vi "test_FHWM.vi"() -> ()   [LabVIEW 2010]
uses:
  <userlib>/gfitsio/cfitsio-bitpix.ctl
  <userlib>/gfitsio/gfitsio-write-image-subset-sgl-2d.vi
  <userlib>/gfitsio/gfitsio.lvlib
panel:
  out "standard error":string
  out "standard output":string
  out "Y FWHM":dbl
  out "X FWHM":dbl
  in  "file path":path
  in  "GuidingStar":i32[][](graph)=[[309, 321, 390, 345, 402, 429, 369, 350, 376, 446, 351, 379, 352, 433, 465, 428, 405, 434, 390, 451, 355, 427, 455, 373, 373, 382, 407, 375, 357, 334, 281, 423], [362, 320, 373, 482, 385, 392, 364, 408, 398, 394, 436, 441, 484, 430, 505, 486, 452, 396, 448, 421, 415, 430, 363, 393, 473, 365, 337, 363, 396, 352, 342, 314], [417, 380, 414, 379, 438, 403, 518, 467, 469, 542, 514, 462, 541, 513, 503, 478, 546, 555, 525, 534, 510, 508, 452, 452, 440, 497, 425, 460, 378, 384, 437, 370], [291, 408, 345, 406, 406, 391, 490, 415, 451, 464, 469, 482, 479, 592, 534, 617, 582, 651, 534, 608, 533, 546, 502, 464, 481, 420, 401, 426, 427, 369, 365, 381], [444, 344, 357, 415, 447, 451, 389, 456, 410, 560, 515, 560, 540, 611, 640, 660, 653, 638, 654, 635, 619, 553, 506, 527, 537, 482, 443, 526, 380, 421, 412, 352], [413, 430, 389, 460, 469, 502, 481, 483, 501, 532, 660, 673, 737, 685, 795, 855, 831, 938, 738, 816, 711, 705, 655, 550, 547, 517, 518, 434, 467, 475, 439, 435], [391, 342, 490, 394, 485, 498, 494, 539, 569, 614, 630, 793, 834, 856, 956, 973, 1101, 1011, 1042, 957, 865, 766, 732, 684, 680, 584, 533, 564, 478, 598, 410, 456], [365, 340, 405, 510, 514, 534, 516, 661, 656, 691, 754, 885, 987, 1132, 1170, 1267, 1305, 1364, 1216, 1278, 993, 973, 841, 883, 741, 564, 579, 490, 590, 501, 440, 451], [409, 405, 430, 463, 544, 553, 603, 650, 765, 840, 906, 1134, 1123, 1399, 1536, 1694, 1650, 1728, 1711, 1528, 1303, 1170, 997, 877, 919, 738, 659, 669, 591, 596, 483, 514], [456, 469, 513, 505, 489, 589, 638, 769, 803, 945, 1114, 1345, 1566, 1679, 1933, 2132, 2273, 2098, 2068, 1908, 1615, 1462, 1274, 1103, 1003, 911, 787, 650, 626, 608, 543, 474], [553, 456, 508, 563, 632, 676, 833, 854, 1011, 1212, 1417, 1611, 1915, 2223, 2450, 2772, 2737, 2709, 2664, 2251, 2090, 1849, 1663, 1307, 1106, 1028, 966, 816, 672, 739, 614, 581], [499, 468, 636, 629, 712, 815, 947, 1042, 1154, 1378, 1677, 2096, 2447, 2665, 3210, 3168, 3590, 3328, 3183, 2928, 2561, 2180, 1910, 1680, 1463, 1277, 1172, 1007, 735, 717, 680, 546], [532, 608, 644, 754, 765, 921, 1100, 1193, 1490, 1835, 2067, 2618, 3039, 3363, 3813, 4084, 4036, 4152, 3873, 3698, 3260, 2887, 2285, 2164, 1767, 1349, 1239, 992, 1016, 770, 704, 616], [545, 598, 687, 868, 924, 1142, 1370, 1547, 1804, 2298, 2694, 3242, 3641, 4271, 4657, 4771, 4952, 4816, 4628, 4458, 3938, 3484, 3038, 2517, 2053, 1742, 1306, 1245, 1009, 898, 714, 696], [559, 650, 818, 968, 1124, 1444, 1578, 1866, 2308, 2721, 3414, 3823, 4408, 5004, 5426, 5623, 5761, 5776, 5527, 5021, 4731, 4090, 3562, 2914, 2374, 1883, 1663, 1322, 1176, 986, 831, 760], [608, 674, 909, 963, 1286, 1512, 1892, 2110, 2615, 3290, 3821, 4557, 5162, 5772, 6236, 6343, 6564, 6500, 6335, 5836, 5439, 4635, 3994, 3325, 2738, 2206, 1783, 1547, 1226, 1127, 955, 752], [628, 629, 951, 1114, 1340, 1638, 1953, 2496, 2919, 3427, 4240, 4903, 5684, 6330, 6836, 7005, 7284, 7183, 7003, 6405, 5678, 5220, 4209, 3691, 2888, 2431, 1912, 1475, 1377, 1053, 889, 778], [693, 927, 1027, 1194, 1447, 1798, 2276, 2805, 3146, 4003, 4560, 5170, 6048, 6824, 7151, 7868, 7951, 8060, 7446, 6937, 6257, 5352, 4730, 3641, 2908, 2500, 1999, 1668, 1334, 1220, 893, 824], [739, 912, 1055, 1224, 1543, 1898, 2330, 2681, 3282, 3700, 4371, 5124, 5763, 6375, 6939, 7349, 8007, 8011, 7674, 7105, 6109, 5237, 4287, 3619, 3026, 2396, 2041, 1590, 1349, 1064, 936, 802], [698, 958, 1022, 1307, 1655, 1767, 2188, 2444, 3042, 3508, 4067, 4781, 5413, 6018, 6876, 7370, 7636, 7986, 7494, 6897, 6025, 5016, 4206, 3408, 2832, 2480, 1994, 1696, 1316, 1127, 991, 861], [764, 844, 992, 1181, 1463, 1819, 1955, 2308, 2549, 3134, 3588, 4016, 4469, 5296, 5824, 6396, 6671, 7075, 6764, 6060, 5241, 4325, 3534, 3075, 2654, 2154, 1769, 1614, 1293, 1058, 863, 795], [721, 891, 985, 1213, 1345, 1606, 1783, 1894, 2355, 2742, 2985, 3464, 3807, 4510, 4822, 5505, 5955, 6311, 5876, 5459, 4573, 3862, 3091, 2772, 2328, 1899, 1677, 1382, 1121, 1045, 868, 768], [713, 712, 926, 1009, 1223, 1415, 1635, 1719, 1854, 2313, 2470, 2765, 3087, 3443, 3861, 4219, 4726, 5054, 4905, 4321, 3857, 3158, 2653, 2190, 1875, 1707, 1368, 1286, 1019, 1022, 822, 792], [605, 695, 852, 1003, 1144, 1267, 1404, 1502, 1738, 1812, 2086, 2188, 2583, 2825, 3068, 3468, 3914, 3994, 3962, 3599, 3038, 2630, 2253, 1989, 1683, 1420, 1322, 1172, 1063, 885, 763, 735], [650, 677, 757, 852, 982, 1109, 1125, 1280, 1465, 1533, 1641, 1764, 1954, 2162, 2395, 2527, 2827, 2983, 2977, 2593, 2408, 1931, 1745, 1608, 1401, 1245, 1190, 940, 956, 839, 774, 646], [603, 631, 686, 775, 915, 970, 939, 1135, 1207, 1263, 1369, 1398, 1620, 1731, 1876, 1981, 2188, 2329, 2251, 2053, 1781, 1718, 1479, 1352, 1223, 1149, 1031, 940, 857, 710, 740, 585], [538, 582, 619, 680, 881, 817, 947, 874, 1016, 1012, 1090, 1246, 1272, 1386, 1405, 1547, 1748, 1694, 1614, 1569, 1420, 1320, 1279, 1112, 1023, 948, 896, 848, 778, 631, 630, 627], [513, 506, 626, 636, 626, 816, 784, 809, 828, 948, 851, 953, 1064, 1117, 1279, 1239, 1369, 1347, 1422, 1252, 1300, 1089, 1093, 984, 953, 934, 803, 721, 667, 586, 623, 632], [411, 540, 502, 700, 642, 602, 633, 654, 712, 692, 757, 802, 804, 926, 968, 959, 1019, 1138, 990, 1126, 938, 931, 871, 790, 731, 695, 673, 746, 594, 548, 557, 484], [440, 534, 548, 525, 542, 539, 666, 632, 643, 735, 662, 689, 671, 803, 866, 872, 767, 918, 825, 884, 777, 784, 751, 810, 736, 696, 624, 665, 627, 598, 493, 512], [402, 410, 454, 489, 454, 623, 560, 571, 563, 617, 550, 588, 695, 623, 683, 656, 678, 726, 719, 713, 635, 703, 636, 701, 669, 579, 672, 482, 577, 514, 475, 445], [416, 371, 456, 445, 450, 461, 512, 467, 478, 520, 506, 596, 569, 604, 575, 643, 623, 566, 596, 624, 660, 595, 565, 566, 577, 532, 545, 520, 466, 468, 450, 457]]
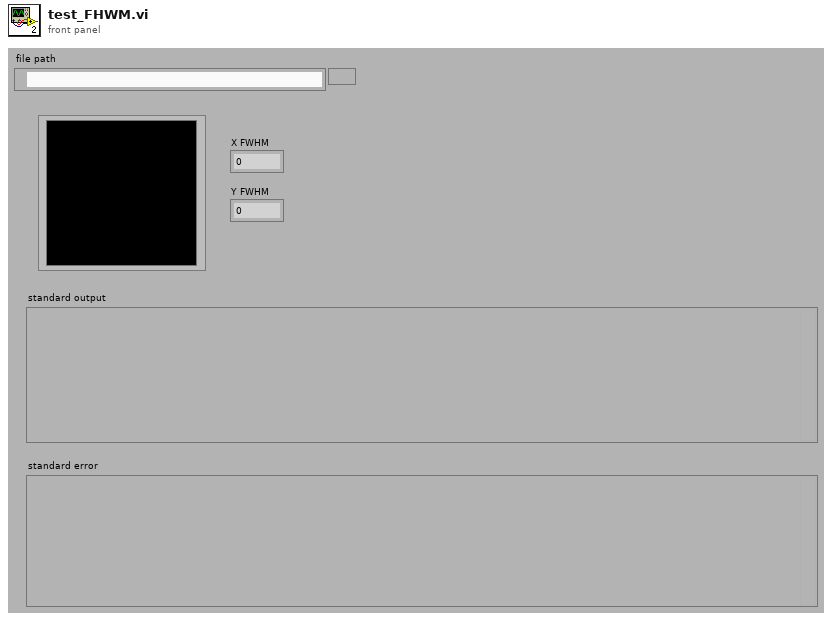
[diagram p1: front panel]
types:
  T1 = enum16{"open", "open or create", "create", "create or replace"}
  T2 = enum16{"open", "open or create", "create or replace", "create", "open (read only)"}
  T3 = typedef "gfitsio.lvlib/cfitsio-bitpix.ctl" = i32
  T4 = typedef "gfitsio.lvlib/gfitsio-refnum.ctl" = refnum<k1>
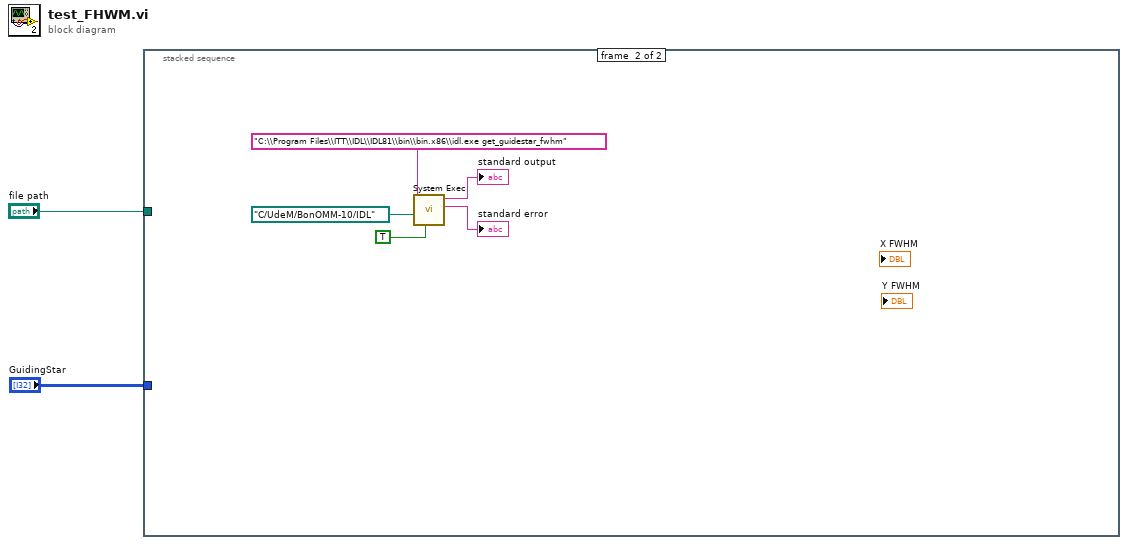
[diagram p0: block diagram]
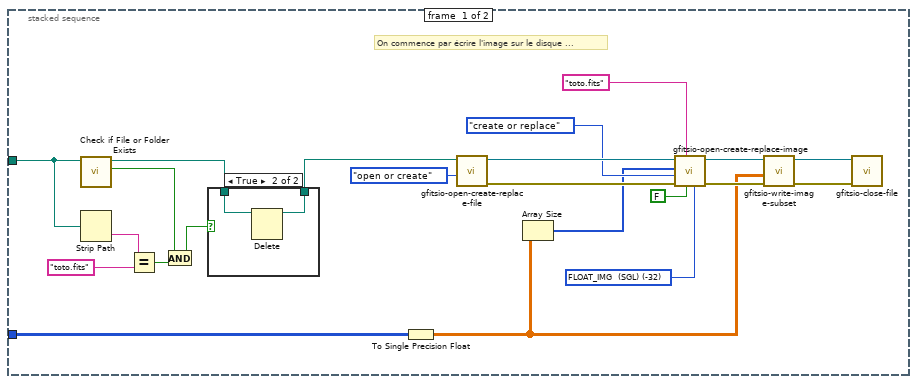
[diagram p2: hidden frame]
diagram:
  n1 = stacked-sequence {
    tunnel: "GuidingStar" -> [w24 _]
    tunnel: "file path" -> [w19 _]
    frame #0 {
      w5 = T3 -32 items=["<invalid type>"=0, "BYTE_IMG  (U8)"=8, "SHORT_IMG  (I16)"=16, "USHORT_IMG  (U16)"=20, "LONG_IMG  (I32)"=32, "ULONG_IMG  (U32)"=40, "FLOAT_IMG  (SGL)"=-32, "DOUBLE_IMG  (DBL)"=-64] ("image data type")
      # "On commence par écrire l'image sur le disque ..."
      n2 = call <vilib>:"Check if File or Folder Exists.vi"("path"=w19) -> ("file or folder exists?"=w14:bool, "dup path"=w21:path)  [unwired: 8 in, 1 out]
      n3 = Strip Path(path=w19) -> (name=w17:string)  [unwired: 1 out]
      n4 = Equal?(x=w17, y="toto.fits") -> (x = y?=w18:bool)
      n5 = And(x=w14, y=w18) -> (x .and. y?=w15:bool)
      n6 = case shown="True" w15 {
        tunnel: w21 -> [w25 w27]
        tunnel: [w25 w26] -> w20
        frame False {
        }
        frame True {
          n7 = Delete(path (use dialog)=w27) -> (deleted path=w26:path)  [unwired: 4 in, 2 out]
        }
      }
      n8 = To Single Precision Float(number=w24) -> (single precision float=w4:sgl[][])
      n9 = call <userlib>:"gfitsio-open-create-replace-file.vi"("function (open)"=T2."open or create", "file path (dialog if empty)"=w20) -> ("error out"=w11:errorcluster, "gfits refnum"=w12:T4)  [unwired: 7 in, 1 out]
      n10 = Array Size(array=w4) -> (size(s)=w3:i32[])
      n11 = call <userlib>:"gfitsio-open-create-replace-image.vi"("image data type"=w5, "advisory dialog? (display:T)"=FALSE, "hdu name (dialog if empty)"="toto.fits", "error in (no error)"=w11, "function (open or create)"=T1."create or replace", "naxes"=w3, "gfits refnum"=w12) -> ("error out"=w10:errorcluster, "dup gfits refnum"=w9:T4)  [unwired: 2 in, 1 out]
      n12 = call-poly <userlib>:"gfitsio-write-image-subset.vi"("error in (no error)"=w10, "data"=w4, "gfits refnum"=w9) -> ("error out"=w22:errorcluster, "dup gfits refnum"=w23:T4)  [unwired: 7 in]
      n13 = call <userlib>:"gfitsio-close-file.vi"("error in (no error)"=w22, "gfits refnum"=w23) -> ()  [unwired: 8 in, 2 out]
    }
    frame #1 {
      n14 = call <vilib>:"System Exec.vi"("run minimized? (F)"=TRUE, "working directory"=path "C:/UdeM/BonOMM-10/IDL" ("command line"), "command line"="C:\\Program Files\\ITT\\IDL\\IDL81\\bin\\bin.x86\\idl.exe get_guidestar_fwhm") -> ("standard error"=→"standard error":string, "standard output"=→"standard output":string)  [unwired: 5 in, 2 out]
    }
  }
